vi "transmitRFID - Copy.vi"() -> ()   [LabVIEW 2015]
uses:
  <instrlib>/niUSRP/niUSRP Write Tx Data (CDB).vi
panel:
  in  "Bandwidth":dbl
  out "coerced bandwidth":dbl
  out "Waveform Phase":dbl[](graph)
  out "Waveform Magnitude":dbl[](graph)
  out "Samples":i32
  out "Loop":i32
  in  "Symbol Rate [Hz]":dbl=10000000.0 format="%#_13p"
  in  "Parameters Select":T1={"Target"=7, "Action"=0, "MemBank"=1, "truncate"=FALSE} {"MemBank" items=["00 RFU", "01 EPC", "10 TID", "11 User"]; "Action" items=["000", "001", "010", "011", "100", "101", "110", "111"]; "Target" items=["000 Inventoried (S0)", "001 Inventoried (S1)", "010 Inventoried (S2)", "011 Inventoried (S3)", "100 SL", "101 RFU", "110 RFU", "111 RFU"]}
  in  "Parameters Symbols":T2={"Tari"=2.5e-05, "PW"=0.5, "factor for \"1\" symbol"=0.5, "RTcal"=2.5, "TRcal"=2.5, "Delimiter"=1.25e-05} {"TRcal" min=1.1 max=3.0 step=0.1; "RTcal" min=2.5 max=3.0 step=0.1; "factor for \"1\" symbol" min=0.5 max=1.0 step=0.1; "PW" min=0.265 max=0.525 step=0.001; "Tari" format="%#_3p"}
  out "coerced IQ rate":dbl=100000.0 format="%#_6p"
  out "carrier frequency":dbl=100000.0 format="%#_6p"
  out "coerced gain":dbl format="%#_6f"
  out "error out":errorcluster
  in  "stop":bool
  in  "IQ rate":dbl=100000.0 format="%#_6p"
  in  "carrier frequency":dbl=100000.0 format="%#_6p"
  in  "gain":dbl format="%#_6f"
  in  "tx device names":refnum<k15>
  # "Transmit RFID"
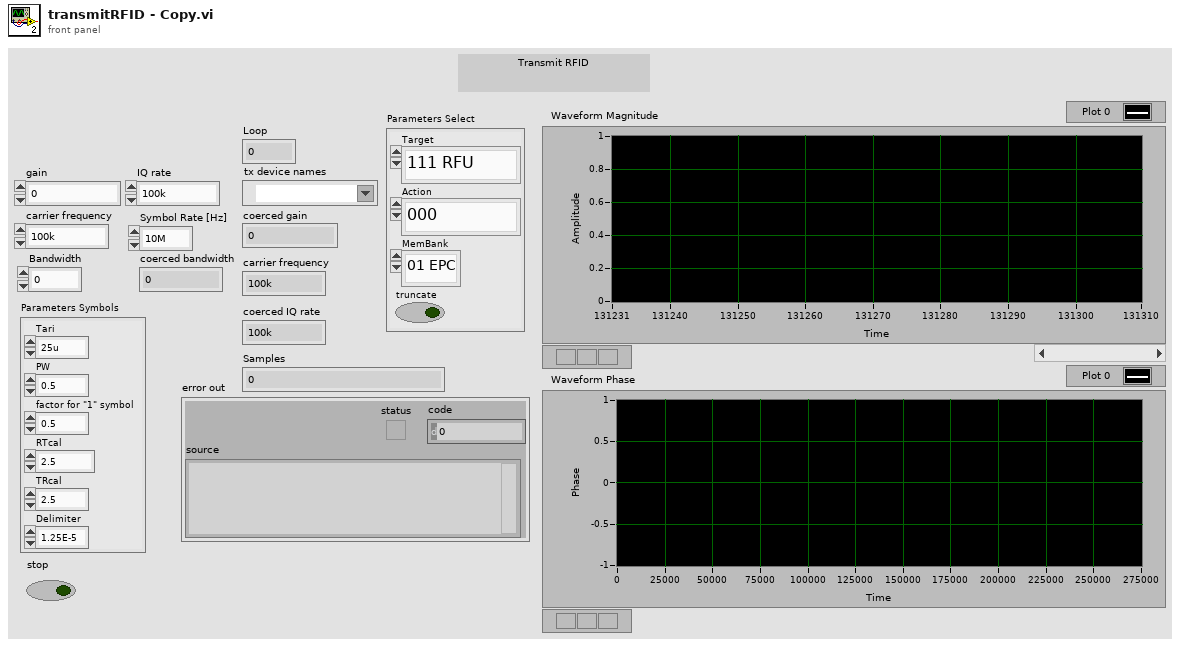
[diagram p1: front panel]
types:
  T1 = cluster{"Target":u16, "Action":u16, "MemBank":u16, "truncate":bool}
  T2 = cluster{"Tari":dbl, "PW":dbl, "factor for \"1\" symbol":dbl, "RTcal":dbl, "TRcal":dbl, "Delimiter":dbl}
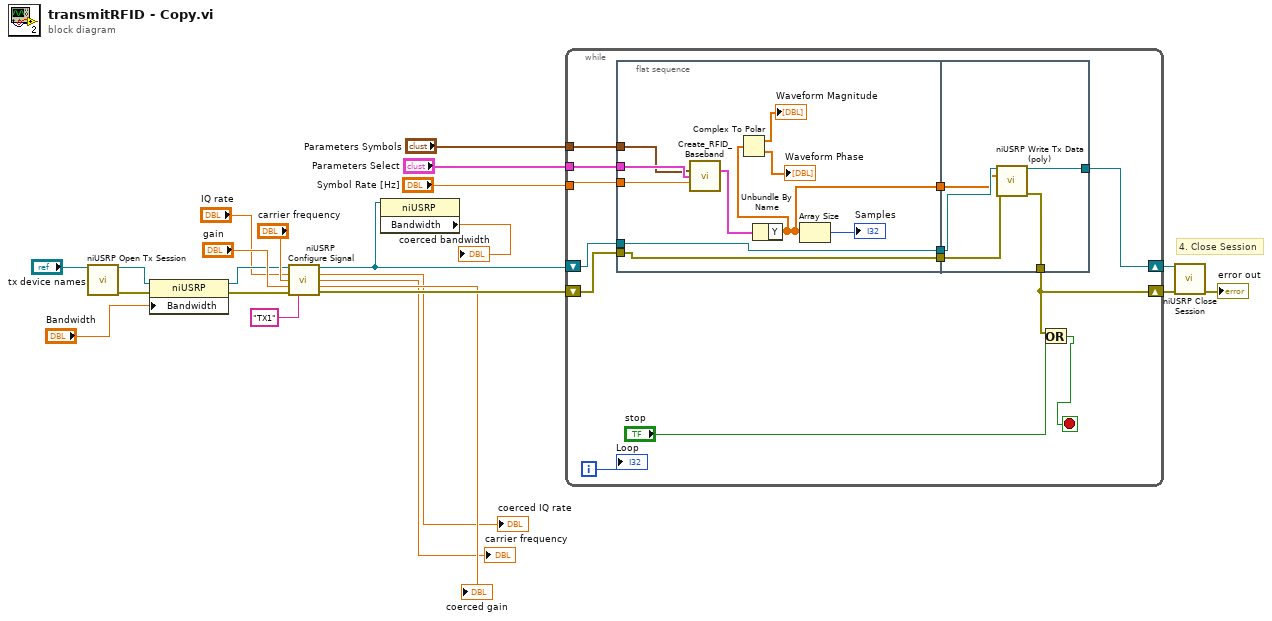
[diagram p0: block diagram]
diagram:
  # "4. Close Session"
  n1 = call <instrlib>:"niUSRP Open Tx Session.vi"("device names"="tx device names") -> ("session handle out"=w5:refnum<k15>, "error out"=w4:errorcluster)  [unwired: 13 in]
  n2 = property class="niUSRP"(reference=w5, error in=w4, "Bandwidth"="Bandwidth") -> (reference out=w6:refnum<k15>, error out=w3:errorcluster)
  n3 = call <instrlib>:"niUSRP Configure Signal.vi"("session handle"=w6, "IQ rate"="IQ rate", "carrier frequency"="carrier frequency", "gain"="gain", "error in (no error)"=w3, "active antenna"="TX1") -> ("session handle out"=w7:refnum<k15>, "coerced IQ rate"=→"coerced IQ rate":dbl, "coerced carrier frequency"=→"carrier frequency":dbl, "coerced gain"=→"coerced gain":dbl, "error out"=w19:errorcluster)  [unwired: 5 in]
  n4 = property class="niUSRP"(reference=w7) -> ("Bandwidth"=→"coerced bandwidth":dbl)  [unwired: 1 in, 2 out]
  n5 = while {
    shift-right: [w29] -> w18
    shift-left: w7 -> [w26]
    shift-right: [w28] -> w17
    shift-left: w19 -> [w25]
    tunnel: "Parameters Symbols" -> [w30]
    tunnel: "Parameters Select" -> [w31]
    tunnel: "Symbol Rate [Hz]" -> [w32]
    i -> [w33]
    stop <- w35 stop-if-true
    n6 = flat-sequence {
      tunnel: w32 -> [w42]
      tunnel: w31 -> [w41]
      tunnel: w30 -> [w40]
      tunnel: [w39] -> w27
      tunnel: w26 -> [w39]
      tunnel: w25 -> [w38]
      tunnel: [w38] -> w24
      tunnel: [w37] -> w23
      tunnel: [w50] -> w29
      tunnel: [w49] -> w28
      tunnel: w27 -> [w48]
      tunnel: w24 -> [w47]
      tunnel: w23 -> [w46]
      frame #0 {
        n7 = call "Create_RFID_Baseband.vi"("Parameters Symbols"=w40, "Parameters Select"=w41, "Symbol Rate [Hz]"=w42) -> ("output complex waveform"=w36:cluster{"t0":dbl, "dt":dbl, "Y":cdb[]})  [unwired: 11 in, 1 out]
        n8 = Unbundle By Name(w36) -> ("Y"=w37:cdb[])
        n9 = Complex To Polar(r * e^(i*theta)=w37) -> (r=→"Waveform Magnitude":dbl[], theta=→"Waveform Phase":dbl[])
        n10 = Array Size(array=w37) -> (size(s)=→"Samples":i32)
      }
      frame #1 {
        n11 = call-poly <instrlib>:"niUSRP Write Tx Data (poly).vi"("session handle"=w48, "data"=w46, "error in (no error)"=w47) -> ("session handle out"=w50:refnum<k15>, "error out"=w49:errorcluster)  [unwired: 11 in]
      }
    }
    n12 = Or(x=w28, y="stop") -> (x .or. y?=w35:bool)
    "Loop" <- w33
  }
  n13 = call <instrlib>:"niUSRP Close Session.vi"("session handle"=w18, "error in (no error)"=w17) -> ("error out"=→"error out":errorcluster)  [unwired: 13 in]
